vi "Teardown.vi"(8 "Error in":errorcluster, 9 "Teardown Location":T1, 10 "Unheard Msgs":refnum<class "Msg.lvclass">[](array[class]), 11 "Base Actor in":refnum<class "Base Actor.lvclass">) -> (3 "Base Actor out":refnum<class "Base Actor.lvclass">)   [LabVIEW 2025, in "jettl.lvlib" / "Base Actor.lvlib" / "Base Actor.lvclass"]
uses:
  Base Actor.lvclass
  Teardown Location.ctl
  Msg/Msg.lvclass
  Base Actor.lvclass/Base Actor.ctl
  jettl.lvlib
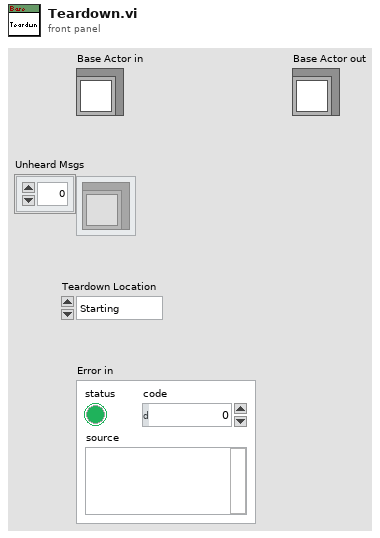
[diagram p1: front panel]
types:
  T1 = typedef "jettl.lvlib/Teardown Location.ctl" = enum16{"Starting", "Stopping"}
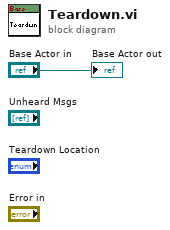
[diagram p0: block diagram]
diagram:
  "Base Actor out" <- "Base Actor in"
